vi "LWXPS_PositionerFeedforwardAccGet.vi"(0 "XPS Reference IN":refnum<k24>, 2 "Positioner Name":string, 5 "LabVIEW error IN":errorcluster) -> (12 "XPS Reference OUT":refnum<k24>, 13 "LabVIEW error OUT":errorcluster, 14 "Returned error code":i32, 15 "Output Name 1":string, 16 "Scale 1":dbl, 17 "Output Name 2":string, 18 "Scale 2":dbl, 19 "XPS Error String":string)   [LabVIEW 2014]
uses:
  D:/XPSQ8_LabView_Library/Development/Source/Dll/Newport.XPS.CommandInterface.dll
  Dll/Newport.XPS.CommandInterface.dll
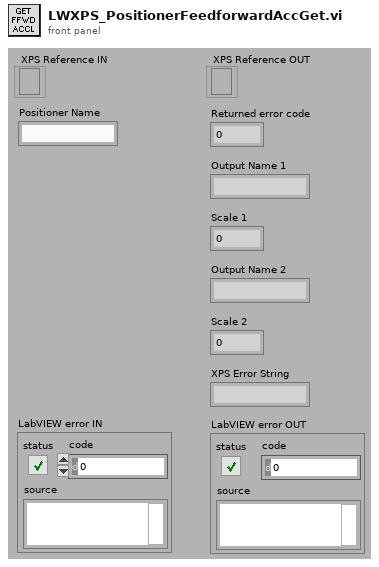
[diagram p1: front panel]
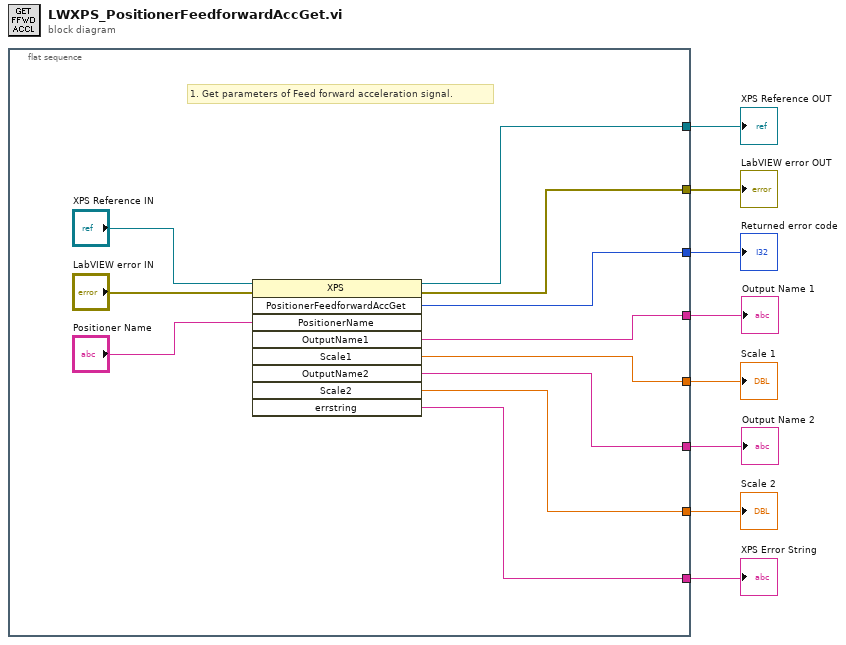
[diagram p0: block diagram]
diagram:
  n1 = flat-sequence {
    tunnel: [w17] -> w8
    tunnel: [w15] -> w7
    tunnel: [w18] -> w6
    tunnel: [w10] -> w2
    tunnel: [w14] -> w5
    tunnel: [w13] -> w1
    tunnel: [w12] -> w3
    tunnel: [w11] -> w4
    frame #0 {
      # "1. Get parameters of Feed forward acceleration signal."
      n2 = invoke class="XPS" method="PositionerFeedforwardAccGet"(reference="XPS Reference IN", error in="LabVIEW error IN", "PositionerName"="Positioner Name") -> (reference out=w17:refnum<k24>, error out=w15:errorcluster, "PositionerFeedforwardAccGet"=w18:i32, "OutputName1"=w10:string, "Scale1"=w14:dbl, "OutputName2"=w13:string, "Scale2"=w12:dbl, "errstring"=w11:string)  [unwired: 6 in, 1 out]
    }
  }
  "XPS Error String" <- w4
  "XPS Reference OUT" <- w8
  "LabVIEW error OUT" <- w7
  "Returned error code" <- w6
  "Scale 1" <- w5
  "Scale 2" <- w3
  "Output Name 1" <- w2
  "Output Name 2" <- w1
